vi "Destroy DS Alert.vi"(8 "error in (no error)":errorcluster, 11 "handle":i64) -> (0 "error out":errorcluster)   [LabVIEW 2026, in "MrcLib.lvlib"]
doc: "Destroy and free any memory associated with the Alert."
uses:
  MrcLib.lvlib
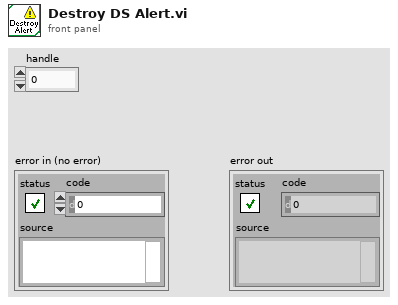
[diagram p1: front panel]
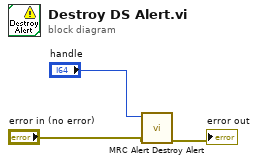
[diagram p0: block diagram]
diagram:
  n1 = call "MRC Alert Destroy Alert.vi"("error in (no error)"="error in (no error)", "handle"="handle") -> ("error out"=→"error out":errorcluster)  [unwired: 9 in]
